vi "bats.parser.test.AddOrderLong.add.two.tickers.vi"(10 "Expected OrderBook.Command[]":T2[](array[typedef])=[{"OrderBook Command.Type"=enum."AddOrder", "Side (U8)"=66, "Order Id (U64)"=3544385890602799695, "Quantity (U32)"=20000, "Symbol (U64)"=4702127773838221344, "Price (U64)"=9050, "Executed Quantity (U32)"=0, "Canceled Quantity (U32)"=0, "Remaining Quantity (U32)"=0, "Seconds (U64)"=0, "Nanoseconds (U64)"=447001}, {"OrderBook Command.Type"=enum."AddOrder", "Side (U8)"=66, "Order Id (U64)"=3616443484640727631, "Quantity (U32)"=20001, "Symbol (U64)"=4702127773838221344, "Price (U64)"=9050, "Executed Quantity (U32)"=0, "Canceled Quantity (U32)"=0, "Remaining Quantity (U32)"=0, "Seconds (U64)"=0, "Nanoseconds (U64)"=447002}, {"OrderBook Command.Type"=enum."AddOrder", "Side (U8)"=66, "Order Id (U64)"=3688501078678655567, "Quantity (U32)"=20002, "Symbol (U64)"=6076284164848492576, "Price (U64)"=9050, "Executed Quantity (U32)"=0, "Canceled Quantity (U32)"=0, "Remaining Quantity (U32)"=0, "Seconds (U64)"=0, "Nanoseconds (U64)"=447003}, {"OrderBook Command.Type"=enum."AddOrder", "Side (U8)"=66, "Order Id (U64)"=3760558672716583503, "Quantity (U32)"=20000, "Symbol (U64)"=4702127773838213120, "Price (U64)"=9050, "Executed Quantity (U32)"=0, "Canceled Quantity (U32)"=0, "Remaining Quantity (U32)"=0, "Seconds (U64)"=0, "Nanoseconds (U64)"=0}, {"OrderBook Command.Type"=enum."AddOrder", "Side (U8)"=66, "Order Id (U64)"=3832616266754511439, "Quantity (U32)"=20000, "Symbol (U64)"=4702127773838213120, "Price (U64)"=9050, "Executed Quantity (U32)"=0, "Canceled Quantity (U32)"=0, "Remaining Quantity (U32)"=0, "Seconds (U64)"=0, "Nanoseconds (U64)"=0}, {"OrderBook Command.Type"=enum."AddOrder", "Side (U8)"=66, "Order Id (U64)"=3904673860792439375, "Quantity (U32)"=20000, "Symbol (U64)"=4702127773838213120, "Price (U64)"=9050, "Executed Quantity (U32)"=0, "Canceled Quantity (U32)"=0, "Remaining Quantity (U32)"=0, "Seconds (U64)"=0, "Nanoseconds (U64)"=0}, {"OrderBook Command.Type"=enum."AddOrder", "Side (U8)"=66, "Order Id (U64)"=3976731454830367311, "Quantity (U32)"=20000, "Symbol (U64)"=4702127773838213120, "Price (U64)"=9050, "Executed Quantity (U32)"=0, "Canceled Quantity (U32)"=0, "Remaining Quantity (U32)"=0, "Seconds (U64)"=0, "Nanoseconds (U64)"=0}, {"OrderBook Command.Type"=enum."AddOrder", "Side (U8)"=66, "Order Id (U64)"=4048789048868295247, "Quantity (U32)"=20000, "Symbol (U64)"=4702127773838213120, "Price (U64)"=9050, "Executed Quantity (U32)"=0, "Canceled Quantity (U32)"=0, "Remaining Quantity (U32)"=0, "Seconds (U64)"=0, "Nanoseconds (U64)"=0}, {"OrderBook Command.Type"=enum."AddOrder", "Side (U8)"=66, "Order Id (U64)"=4120846642906223183, "Quantity (U32)"=20000, "Symbol (U64)"=4702127773838213120, "Price (U64)"=9050, "Executed Quantity (U32)"=0, "Canceled Quantity (U32)"=0, "Remaining Quantity (U32)"=0, "Seconds (U64)"=0, "Nanoseconds (U64)"=0}, {"OrderBook Command.Type"=enum."AddOrder", "Side (U8)"=66, "Order Id (U64)"=4697307395209646671, "Quantity (U32)"=20000, "Symbol (U64)"=4702127773838213120, "Price (U64)"=9050, "Executed Quantity (U32)"=0, "Canceled Quantity (U32)"=0, "Remaining Quantity (U32)"=0, "Seconds (U64)"=0, "Nanoseconds (U64)"=0}, {"OrderBook Command.Type"=enum."AddOrder", "Side (U8)"=66, "Order Id (U64)"=4769364989247574607, "Quantity (U32)"=20000, "Symbol (U64)"=4702127773838213120, "Price (U64)"=9050, "Executed Quantity (U32)"=0, "Canceled Quantity (U32)"=0, "Remaining Quantity (U32)"=0, "Seconds (U64)"=0, "Nanoseconds (U64)"=0}] {"Side (U8)" format="%.0x"; "Order Id (U64)" format="%.0x"; "Symbol (U64)" format="%.0x"}) -> ()   [LabVIEW 2022 SP3]
uses:
  fpga/common/orderbook.command.ctl
  fpga/common/orderbook.command.type.ctl
  pitch/AddOrder/AddOrderLong.Parameters.ctl
  pitch/AddOrder/AddOrderLong.lvclass
panel:
  out "Passed":bool
  in  "AddOrderLong.Parameters 3":T1={"Time Offset"=447003, "Order Id"="ORID0003", "Quantity"=20002, "Symbol"="TSLA", "Side Indicator"="B", "Price"=0.905}
  in  "AddOrderLong.Parameters 2":T1={"Time Offset"=447002, "Order Id"="ORID0002", "Quantity"=20001, "Symbol"="AAPL", "Side Indicator"="B", "Price"=0.905}
  in  "AddOrderLong.Parameters":T1={"Time Offset"=447001, "Order Id"="ORID0001", "Quantity"=20000, "Symbol"="AAPL", "Side Indicator"="B", "Price"=0.905}
  out "Debug":u64[](array[numeric]) format="%.0x"
  out "Results":T2[](array[typedef]) {"Side (U8)" format="%.0x"; "Order Id (U64)" format="%.0x"; "Symbol (U64)" format="%.0x"}
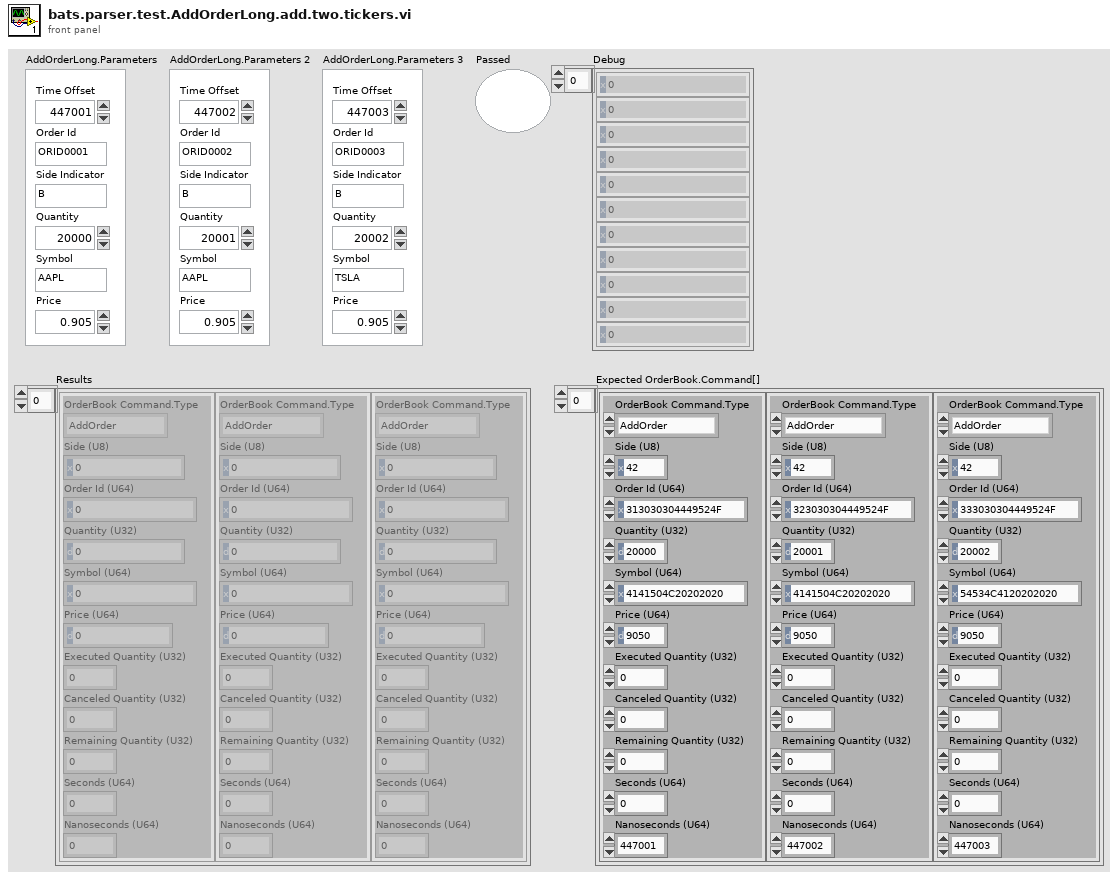
[diagram p1: front panel]
types:
  T1 = typedef "AddOrderLong.lvclass/AddOrderLong.Parameters.ctl" = cluster{"Time Offset":u32, "Order Id":string, "Quantity":u32, "Symbol":string, "Side Indicator":string, "Price":dbl}
  T2 = typedef "orderbook.command.ctl" = cluster{"OrderBook Command.Type":T3, "Side (U8)":u8, "Order Id (U64)":u64, "Quantity (U32)":u32, "Symbol (U64)":u64, "Price (U64)":u64, "Executed Quantity (U32)":u32, "Canceled Quantity (U32)":u32, "Remaining Quantity (U32)":u32, "Seconds (U64)":u64, "Nanoseconds (U64)":u64}
  T3 = typedef "orderbook.command.type.ctl" = enum16{"Time", "AddOrder", "OrderExecuted", "OrderExecutedAtPrice", "ReduceSize", "ModifyOrder", "DeleteOrder", "Get.State", "Get.All.Orders", "Get.Top"}
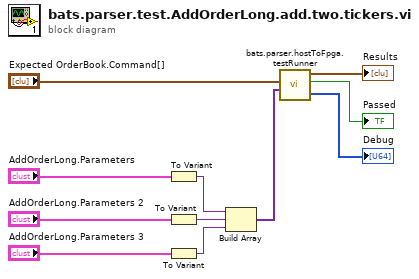
[diagram p0: block diagram]
diagram:
  n1 = To Variant(anything="AddOrderLong.Parameters") -> (Variant=w2:variant)
  n2 = To Variant(anything="AddOrderLong.Parameters 2") -> (Variant=w3:variant)
  n3 = To Variant(anything="AddOrderLong.Parameters 3") -> (Variant=w4:variant)
  n4 = Build Array(w2, w3, w4) -> (w1:variant[])
  n5 = call "bats.parser.hostToFpga.testRunner.vi"("Test.Messages"=w1, "Expected OrderBook.Command[]"="Expected OrderBook.Command[]") -> ("Passed"=→"Passed":bool, "OrderBook.Command[]"=→"Results":T2[], "Debug"=→"Debug":u64[])  [unwired: 6 in, 1 out]
